vi "Set Level.vi"(8 "error in":errorcluster, 10 "Level":T1, 11 "Handler in":refnum<class "Handler.lvclass">) -> (0 "error out":errorcluster, 3 "Handler out":refnum<class "Handler.lvclass">)   [LabVIEW 2024, in "hse-logger.lvlib" / "Handler.lvclass"]
doc: "Sets the log-level of the handler.\n\n____\nHAMPEL SOFTWARE ENGINEERING v2.2.2 (2025-01-16 15:41)"
uses:
  <vilib>/Hampel Software Engineering/HSE Logger/Handler/Handler.lvclass
  <vilib>/Hampel Software Engineering/HSE Logger/LogLevel.ctl
  <vilib>/Hampel Software Engineering/HSE Logger/Handler/Handler.lvclass/Handler.ctl
  <vilib>/Hampel Software Engineering/HSE Logger/hse-logger.lvlib
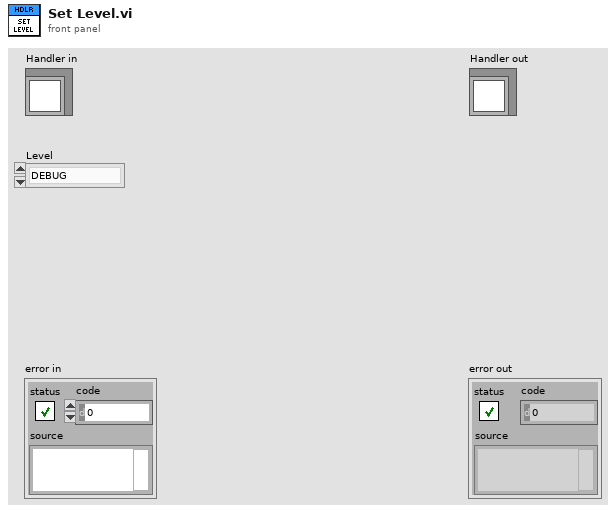
[diagram p1: front panel]
types:
  T1 = typedef "hse-logger.lvlib/LogLevel.ctl" = enum16{"DEBUG", "INFO", "WARNING", "ERROR", "CRITICAL"}
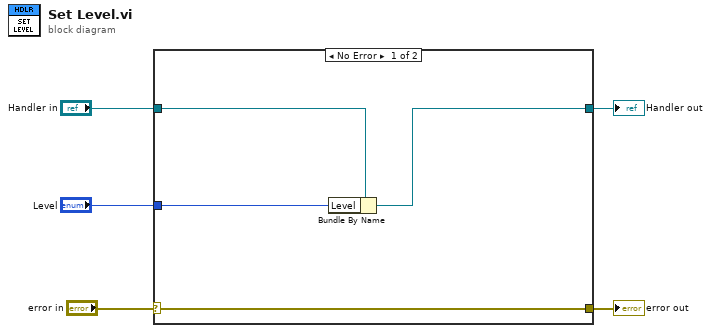
[diagram p0: block diagram]
diagram:
  n1 = case shown="No Error" "error in" {
    selector: "error in" -> [w9 w11]
    tunnel: [w9 w11] -> w4
    tunnel: [w7 w10] -> w2
    tunnel: "Handler in" -> [w8 w10]
    tunnel: "Level" -> [w6 _]
    frame No Error {
      n2 = Bundle By Name(cluster=w8, "Level"=w6) -> (w7:refnum<class "Handler.lvclass">)
    }
    frame Error {
    }
  }
  "error out" <- w4
  "Handler out" <- w2
